vi "OpenPrefDialog.vi"(8 "error in (no error)":errorcluster, 9 "PluginIniFilePath":path, 10 "Class Path":path) -> (0 "error out":errorcluster)   [LabVIEW 2018, in "AnalysisPlugins.lvlib" / "AnalysisPluginsBase.lvclass"]
uses:
  AnalysisPluginsBase.lvclass
  C:/Program Files (x86)/National Instruments/LabVIEW 2018/user.lib/NIST/BaseClasses/BasePlugin_class/BasePlugin.lvclass
  <userlib>/NIST/BaseClasses/BasePlugin_class/BasePlugin.lvclass/BasePlugin.ctl
  <userlib>/NIST/BaseClasses/BasePlugin_class/Accessors/Write PluginIniFilePath.vi
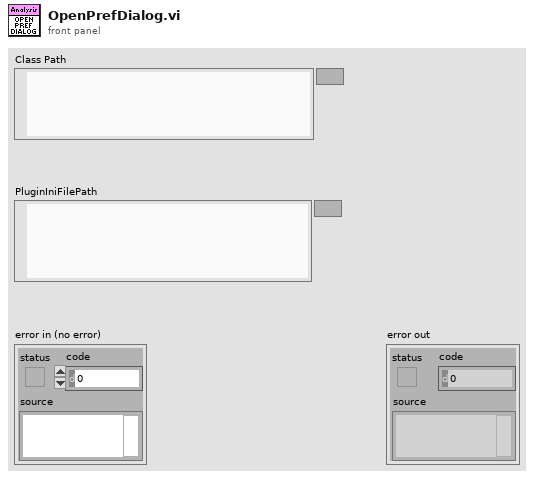
[diagram p1: front panel]
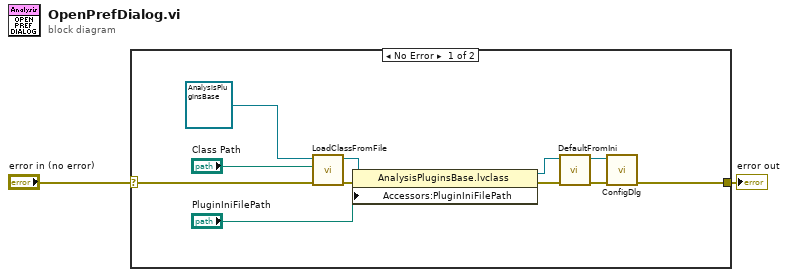
[diagram p0: block diagram]
diagram:
  n1 = case shown="No Error" "error in (no error)" {
    selector: "error in (no error)" -> [w5 w14]
    tunnel: [w7 w14] -> w1
    frame No Error {
      n2 = call-dynamic "LoadClassFromFile.vi"("error in (no error)"=w5, "class path"="Class Path", "reference in"=refnum<class "AnalysisPluginsBase.lvclass"> refnum ("AcPwrBase in")) -> ("error out"=w12:errorcluster, "reference out"=w11:refnum<class "AnalysisPluginsBase.lvclass">)  [unwired: 7 in]
      n3 = property class="AnalysisPluginsBase.lvclass"(reference=w11, error in=w12, "Accessors:PluginIniFilePath"="PluginIniFilePath") -> (reference out=w10:refnum<class "AnalysisPluginsBase.lvclass">, error out=w13:errorcluster)
      n4 = call-dynamic "DefaultFromIni.vi"("error in (no error)"=w13, "AnalysisPluginsBase in"=w10) -> ("error out"=w8:errorcluster, "AnalysisPluginsBase out"=w9:refnum<class "AnalysisPluginsBase.lvclass">)  [unwired: 8 in]
      n5 = call-dynamic "ConfigDlg.vi"("error in (no error)"=w8, "AnalysisPluginsBase in"=w9) -> ("error out"=w7:errorcluster)  [unwired: 7 in, 2 out]
    }
    frame Error {
    }
  }
  "error out" <- w1
